vi "Lakeshore subVI.vi"(5 "Setpoint 2":dbl format="%.4f", 6 "Rate (D) (X.X %)":dbl=120.0 format="%.1f", 7 "Range":u16(ring) items=["Off", "Low (On)", "Medium", "High"], 8 "Reset (I) (XX.X)":dbl=20.0 format="%.1f", 9 "Gain (P) (XX.X)":dbl=50.0 format="%.1f", 10 "error in (no error)":errorcluster, 11 "VISA resource name":refnum<visa-resource-name>) -> (0 "Input B":dbl, 1 "Input A":dbl, 2 "error out":errorcluster, 3 "VISA resource name out":refnum<visa-resource-name>, 4 "Heater 1 (%)":dbl format="%.1f")   [LabVIEW 2012]
uses:
  <instrlib>/Lake Shore 335/Public/Data/Sensor Data (Single Reading).vi
  <instrlib>/Lake Shore 335/Lake Shore 335.lvlib
panel:
  in  "Manual Output":dbl format="%.2f"
  out "Reset (I)":dbl=20.0 format="%.1f"
  out "Gain (P)":dbl=50.0 format="%.1f"
  out "Rate (D)":dbl format="%.1f"
  out "Setpoint":dbl format="%.4f"
  in  "Unit":u16(ring)=1 items=["Kelvin", "Celcius", "Sensor"]
  in  "Unit 2":u16(ring)=1 items=["Kelvin", "Celcius", "Sensor"]
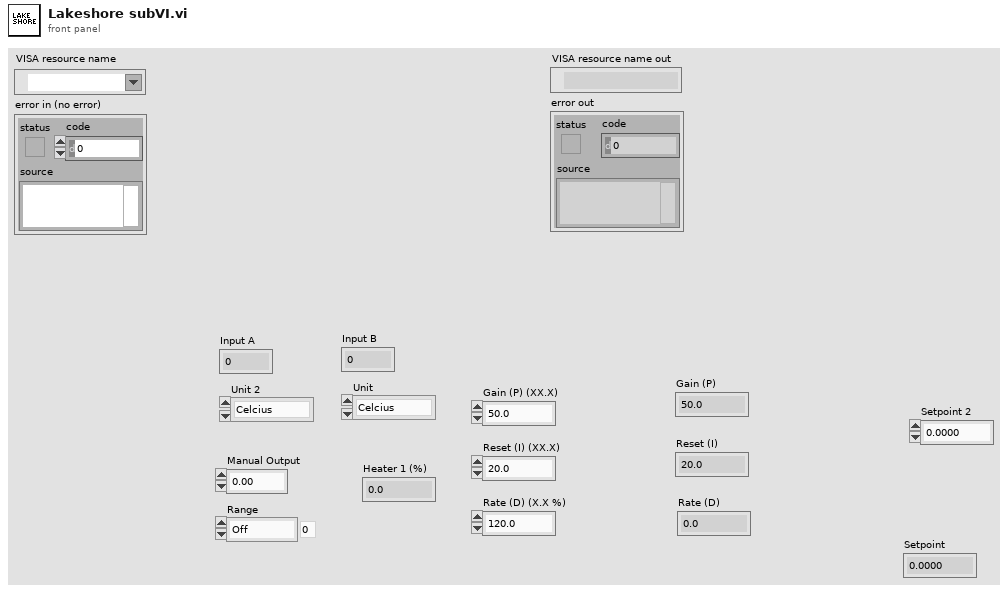
[diagram p1: front panel]
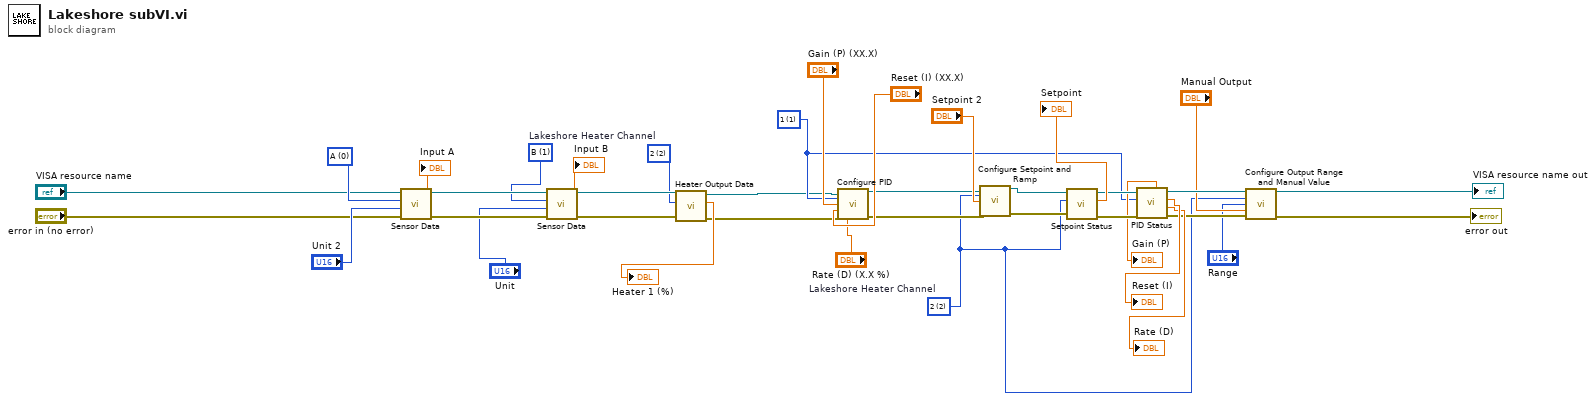
[diagram p0: block diagram]
diagram:
  w8 = u16 2 items=["1"=1, "2"=2]  # Lakeshore Heater Channel
  w7 = u16 1 items=["1"=1, "2"=2] ("Output's Control Loop (1:1)")
  w29 = u16 2 items=["1"=1, "2"=2]  # Lakeshore Heater Channel
  w33 = u16 1 items=["A", "B"] ("Input (0:A)")
  w37 = u16 0 items=["A", "B"] ("Input (0:A)")
  n1 = call-poly <instrlib>:"Sensor Data.vi"("error in (no error)"="error in (no error)", "Data Source (0:Kelvin)"="Unit 2", "Input (0:A)"=w37, "VISA resource name"="VISA resource name") -> ("error out"=w35:errorcluster, "Sensor Data"=→"Input A":dbl, "VISA resource name out"=w36:refnum<visa-resource-name>)  [unwired: 5 in]
  n2 = call-poly <instrlib>:"Sensor Data.vi"("error in (no error)"=w35, "Data Source (0:Kelvin)"="Unit", "Input (0:A)"=w33, "VISA resource name"=w36) -> ("error out"=w30:errorcluster, "Sensor Data"=→"Input B":dbl, "VISA resource name out"=w31:refnum<visa-resource-name>)  [unwired: 5 in]
  n3 = call <instrlib>:"Heater Output Data.vi"("error in (no error)"=w30, "Heater Output (1:1)"=w29, "VISA resource name"=w31) -> ("error out"=w5:errorcluster, "Output Value"=→"Heater 1 (%)":dbl, "VISA resource name out"=w6:refnum<visa-resource-name>)  [unwired: 6 in]
  n4 = call <instrlib>:"Configure PID.vi"("VISA resource name"=w6, "Output's Control Loop (1:1)"=w7, "Gain (P) (50.0)"="Gain (P) (XX.X)", "Reset (I) (20.0)"="Reset (I) (XX.X)", "error in (no error)"=w5, "Rate (D) (0.0 %)"="Rate (D) (X.X %)") -> ("VISA resource name out"=w10:refnum<visa-resource-name>, "error out"=w9:errorcluster)  [unwired: 8 in]
  n5 = call <instrlib>:"Configure Setpoint and Ramp.vi"("VISA resource name"=w10, "Output's Control Loop (1:1)"=w8, "Setpoint (0.0000)"="Setpoint 2", "error in (no error)"=w9) -> ("VISA resource name out"=w25:refnum<visa-resource-name>, "error out"=w24:errorcluster)  [unwired: 10 in]
  n6 = call <instrlib>:"Setpoint Status.vi"("error in (no error)"=w24, "Output (1:1)"=w8, "VISA resource name"=w25) -> ("error out"=w20:errorcluster, "Setpoint"=→"Setpoint":dbl, "VISA resource name out"=w21:refnum<visa-resource-name>)  [unwired: 6 in]
  n7 = call <instrlib>:"PID Status.vi"("error in (no error)"=w20, "Output's Control Loop (1:1)"=w7, "VISA resource name"=w21) -> ("error out"=w15:errorcluster, "Rate (D)"=→"Rate (D)":dbl, "Reset (I)"=→"Reset (I)":dbl, "VISA resource name out"=w16:refnum<visa-resource-name>, "Gain (P)"=→"Gain (P)":dbl)  [unwired: 4 in]
  n8 = call <instrlib>:"Configure Output Range and Manual Value.vi"("VISA resource name"=w16, "Heater Output (1:1)"=w8, "Range (0:Off)"="Range", "Manual Output (0.00 %)"="Manual Output", "error in (no error)"=w15) -> ("VISA resource name out"=→"VISA resource name out":refnum<visa-resource-name>, "error out"=→"error out":errorcluster)  [unwired: 9 in]
